vi "rethinkdb_json_drop.vi"(8 "error in (no error)":errorcluster, 11 "json":string) -> (0 "error out":errorcluster, 3 "id":u64)   [LabVIEW 2017]
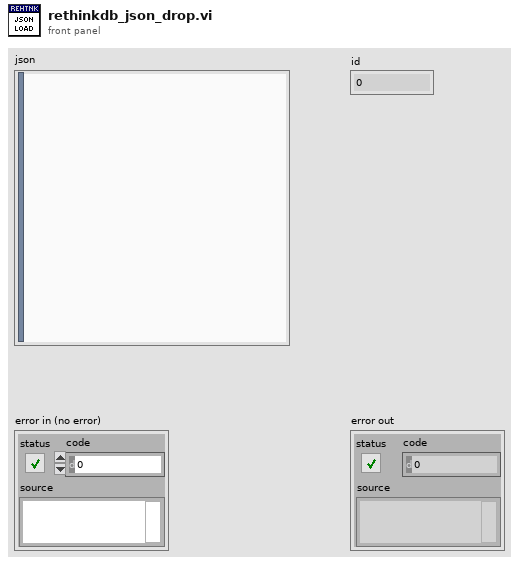
[diagram p1: front panel]
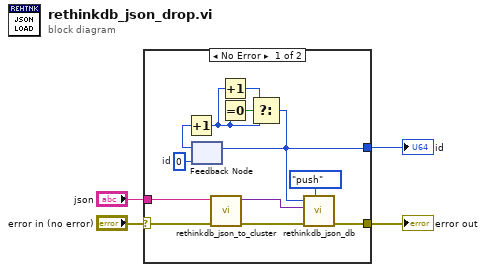
[diagram p0: block diagram]
diagram:
  n1 = case shown="No Error" "error in (no error)" {
    selector: "error in (no error)" -> [w16 w17]
    tunnel: "json" -> [w15 _]
    tunnel: [w5 _] -> w2
    tunnel: [w9 w17] -> w1
    frame No Error {
      w14 = u64 0  # id
      n2 = feedback #1(w14) -> (w13:u64)
      n3 = Increment(x=w13) -> (x+1=w7:u64)
      n4 = call "rethinkdb_json_to_cluster.vi"("error in (no error)"=w16, "json"=w15) -> ("error out"=w12:errorcluster, "cluster"=w11:variant)  [unwired: 7 in, 1 out]
      n5 = Increment(x=w7) -> (x+1=w6:u64)
      n6 = Equal To 0?(x=w7) -> (x = 0?=w8:bool)
      n7 = Select(t=w6, s=w8, f=w7) -> (s? t:f=w5:u64)
      n8 = feedback-in #1(w5) -> ()
      n9 = call "rethinkdb_json_db.vi"("action"=enum8{"get", "push", "pop"}."push", "error in (no error)"=w12, "cluster in"=w11, "id in"=w5) -> ("error out"=w9:errorcluster)  [unwired: 4 in, 3 out]
    }
    frame Error {
    }
  }
  "error out" <- w1
  "id" <- w2
